vi "Append Test Suites to Document.vi"(8 "error in (no error)":errorcluster, 11 "XML Report In":refnum<class "XML Report.lvclass">) -> (0 "error out":errorcluster, 2 "Test Suites Element":refnum<k20>, 3 "XML Report Out":refnum<class "XML Report.lvclass">)   [LabVIEW 2020, in "XML Report.lvclass"]
uses:
  XML Report.lvclass
  <resource>/objmgr/DOMUserDefRef.rc
  Test Report/Test Report.lvclass
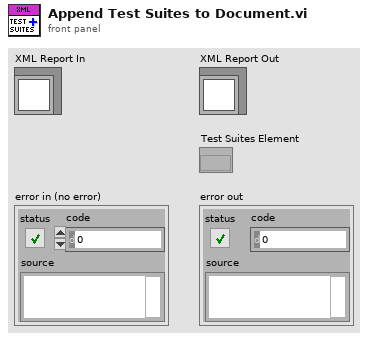
[diagram p1: front panel]
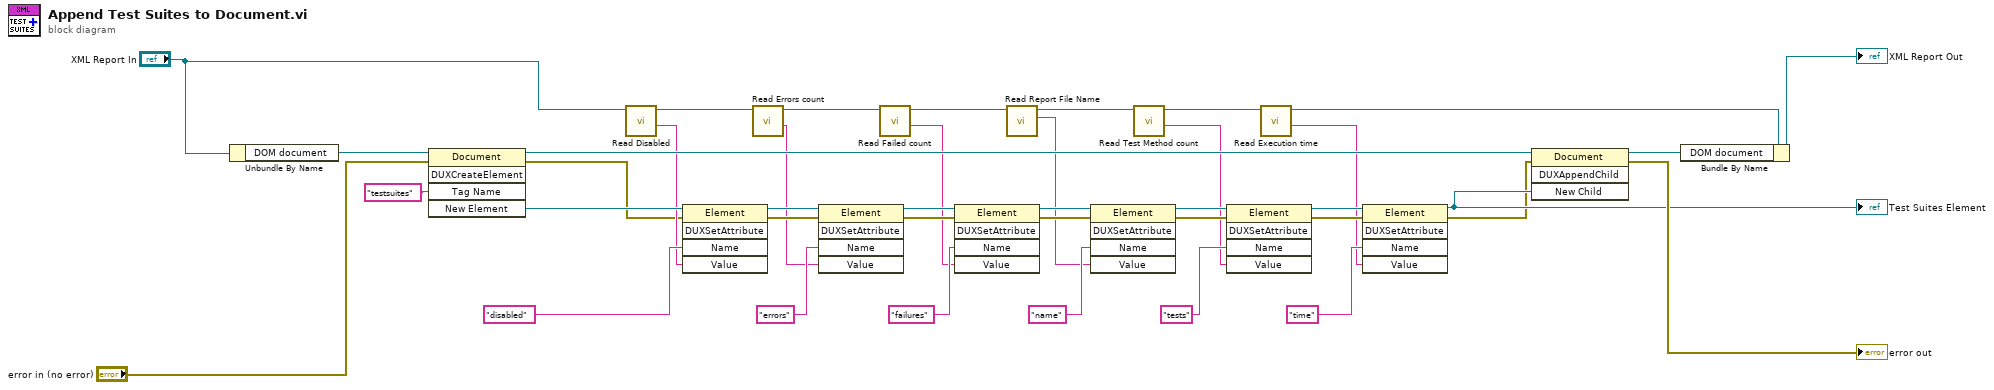
[diagram p0: block diagram]
diagram:
  n1 = Unbundle By Name("XML Report In") -> ("DOM document"=w37:refnum<k20>)
  n2 = invoke class="Document" method="DUXCreateElement"(reference=w37, error in="error in (no error)", "Tag Name"="testsuites") -> (reference out=w36:refnum<k20>, error out=w3:errorcluster, "New Element"=w33:refnum<k20>)  [unwired: 2 in, 2 out]
  n3 = call "Read Disabled.vi"("Report In"="XML Report In") -> ("Disabled string"=w9:string, "Report Out"=w15:refnum<class "XML Report.lvclass">)  [unwired: 7 in, 2 out]
  n4 = invoke class="Element" method="DUXSetAttribute"(reference=w33, error in=w3, "Name"="disabled", "Value"=w9) -> (reference out=w26:refnum<k20>, error out=w25:errorcluster)  [unwired: 1 in, 3 out]
  n5 = call "Read Errors count.vi"("Report In"=w15) -> ("Errors count string"=w4:string, "Report Out"=w14:refnum<class "XML Report.lvclass">)  [unwired: 7 in, 2 out]
  n6 = invoke class="Element" method="DUXSetAttribute"(reference=w26, error in=w25, "Name"="errors", "Value"=w4) -> (reference out=w24:refnum<k20>, error out=w23:errorcluster)  [unwired: 1 in, 3 out]
  n7 = call "Read Failed count.vi"("Report In"=w14) -> ("Failed count string"=w5:string, "Report Out"=w13:refnum<class "XML Report.lvclass">)  [unwired: 7 in, 2 out]
  n8 = invoke class="Element" method="DUXSetAttribute"(reference=w24, error in=w23, "Name"="failures", "Value"=w5) -> (reference out=w22:refnum<k20>, error out=w21:errorcluster)  [unwired: 1 in, 3 out]
  n9 = call-dynamic "Read Report File Name.vi"("XML Report In"=w13) -> ("Report Name"=w6:string, "XML Report Out"=w12:refnum<class "XML Report.lvclass">)  [unwired: 7 in, 2 out]
  n10 = invoke class="Element" method="DUXSetAttribute"(reference=w22, error in=w21, "Name"="name", "Value"=w6) -> (reference out=w20:refnum<k20>, error out=w19:errorcluster)  [unwired: 1 in, 3 out]
  n11 = call "Read Test Method count.vi"("Report In"=w12) -> ("Test Method count string"=w7:string, "Report Out"=w11:refnum<class "XML Report.lvclass">)  [unwired: 7 in, 2 out]
  n12 = invoke class="Element" method="DUXSetAttribute"(reference=w20, error in=w19, "Name"="tests", "Value"=w7) -> (reference out=w18:refnum<k20>, error out=w17:errorcluster)  [unwired: 1 in, 3 out]
  n13 = call "Read Execution time.vi"("Report In"=w11) -> ("Execution time string"=w8:string, "Report Out"=w10:refnum<class "XML Report.lvclass">)  [unwired: 7 in, 2 out]
  n14 = invoke class="Element" method="DUXSetAttribute"(reference=w18, error in=w17, "Name"="time", "Value"=w8) -> (reference out=w2:refnum<k20>, error out=w1:errorcluster)  [unwired: 1 in, 3 out]
  "Test Suites Element" <- w2
  n15 = invoke class="Document" method="DUXAppendChild"(reference=w36, error in=w1, "New Child"=w2) -> (reference out=w39:refnum<k20>, error out=→"error out":errorcluster)  [unwired: 1 in, 2 out]
  n16 = Bundle By Name(cluster=w10, "DOM document"=w39) -> (→"XML Report Out":refnum<class "XML Report.lvclass">)
